vi "Execute_Row.vi"(3 "Simulate/Run":T2, 5 "Traverse line":T3 {"Carrier_2 Q (l/min)" format="%#.2f"; "Row Duration (mins)" format="%#.1f"; "Row No" min=0; "Trace Gas Concentration (%)" min=0.0 format="%#_4f"; "Carrier_1 Q (l/min)" format="%#.4f"; "Start X" format="%#.2f"; "Start Y" format="%#.2f"; "Start Z" format="%#.2f"; "End X" format="%#.2f"; "End Y" format="%#.2f"; "End Z" format="%#.2f"; "Tunnel Speed" format="%#.2f"; "Averaging time (mins)" min=0.0 format="%#.2f"}) -> (1 "Status":T1, 2 "Traverse line out":T3 {"Carrier_2 Q (l/min)" format="%#.2f"; "Row Duration (mins)" format="%#.1f"; "Row No" min=0; "Trace Gas Concentration (%)" min=0.0 format="%#_4f"; "Carrier_1 Q (l/min)" format="%#.4f"; "Start X" format="%#.2f"; "Start Y" format="%#.2f"; "Start Z" format="%#.2f"; "End X" format="%#.2f"; "End Y" format="%#.2f"; "End Z" format="%#.2f"; "Tunnel Speed" format="%#.2f"; "Averaging time (mins)" min=0.0 format="%#.2f"})   [LabVIEW 2021]
uses:
  Traverse_cluster.ctl
  Spacing.ctl
  Controls/Multi_run_mode.ctl
  Controls/User_Specific_mode.ctl
  Multi_Run_Status.ctl
  Controls/Setup.ctl
  Controls/Save_Data.ctl
  Camera Server/Camera enum/Camera resolution.ctl
  ADAM Client/Sub VIs/ADAM Controls/Quick_local_ADAM_Table.ctl
  Globals/Constants_global.vi
  Globals/Extra_Commands_Global.vi
  Globals/Trav_pos_global.vi
panel:
  # "X           Y          Z"
  # "Start"
  # "End"
  # "X           Y          Z"
  # "Start"
  # "End"
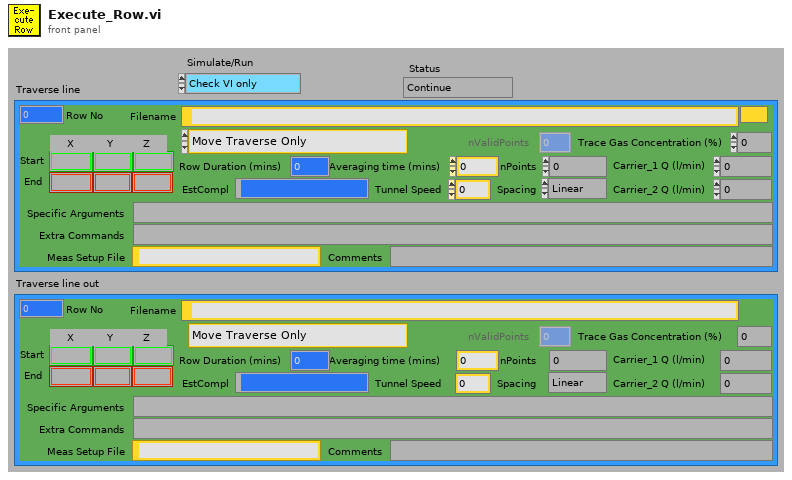
[diagram p1: front panel]
types:
  T1 = typedef "Multi_Run_Status.ctl" = enum16{"Continue", "Continue with Error", "Jump to Next Point", "Jump to Next Row", "Jump To Fall Back", "Terminate Run"}
  T2 = typedef "User_Specific_mode.ctl" = enum16{"Check VI only", "Run VI"}
  T3 = typedef "Traverse_cluster.ctl" = cluster{"Start X":sgl, "Start Y":sgl, "Start Z":sgl, "End X":sgl, "End Y":sgl, "End Z":sgl, "nPoints":i32, "Spacing":T4, "Filename":path, "Tunnel Speed":dbl, "Averaging time (mins)":dbl, "Extra Commands":string, "Carrier_1 Q (l/min)":dbl, "Carrier_2 Q (l/min)":dbl, "Trace Gas Concentration (%)":dbl, "Specific Arguments":string, "Comments":string, "Row No":i32, "Row Type Selector":T5, "EstCompl":string, "Row Duration (mins)":dbl, "nValidPoints":i32, "Meas Setup File":string}
  T4 = typedef "Spacing.ctl" = enum16{"Linear", "Log", "Gauss", "Specified", "N/A"}
  T5 = typedef "Multi_run_mode.ctl" = enum16{"Move Traverse Only", "Set Tunnel Speed Only", "Set Source Only", "Set Measurement Conditions", "Single Measurement", "Vertical Profile", "Lateral Profile", "Longitudinal Profile", "Multi-Axis Profile", "Explore Volume", "Auto Calibrate", "Meas Fast FID Bkgnd", "Check Beam Power", "Scanning Valve Measurement", "Run VI Named:", "Set ADAM Ch", "Wait (minutes)", "Send Message", "Synchronize With:", "Fall Back to this Row", "Turn Off Row Repeating", "Traverse 3D Volume", "Blank Row", "Jump to Fall Back Row"}
  T6 = typedef "Save_Data.ctl" = enum16{"Save No Data", "Save Data"}
  T7 = typedef "Setup.ctl" = enum16{"Run Program", "Show Setup", "Save Current Setup", "Setup Front Panel"}
  T8 = typedef "Quick_local_ADAM_Table.ctl" = enum16{"Read Global", "Load Global From ADAM Table", "Write Global"}
  T9 = typedef "Camera resolution.ctl" = u8
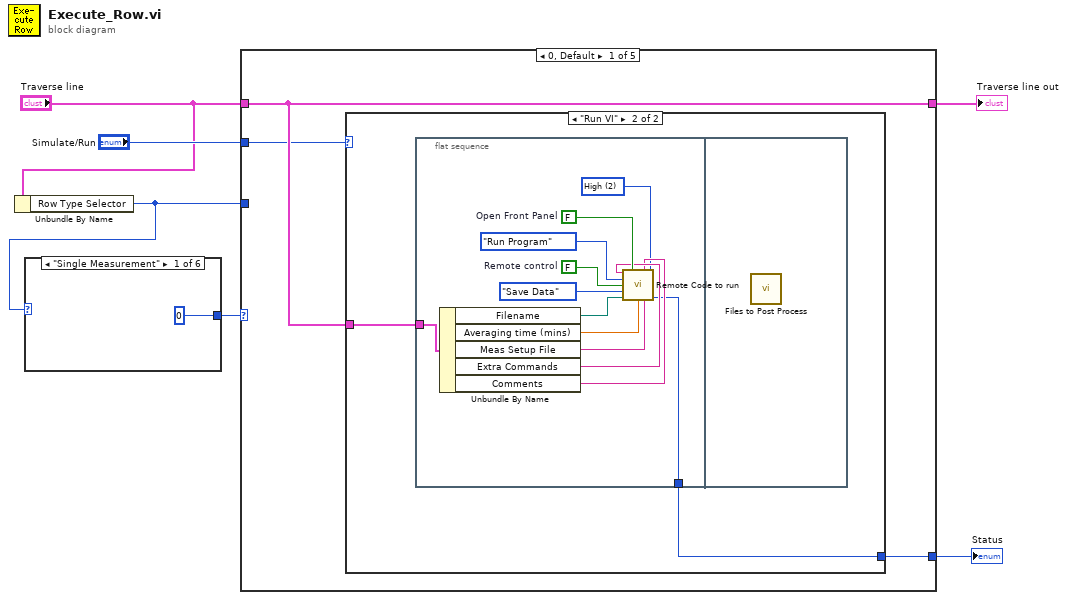
[diagram p0: block diagram]
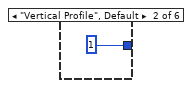
[diagram p2: hidden frame]
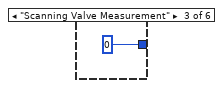
[diagram p3: hidden frame]
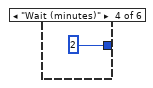
[diagram p4: hidden frame]
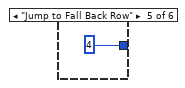
[diagram p5: hidden frame]
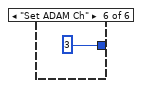
[diagram p6: hidden frame]
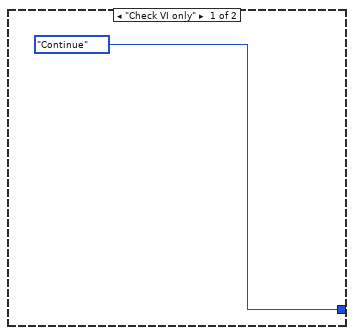
[diagram p7: hidden frame]
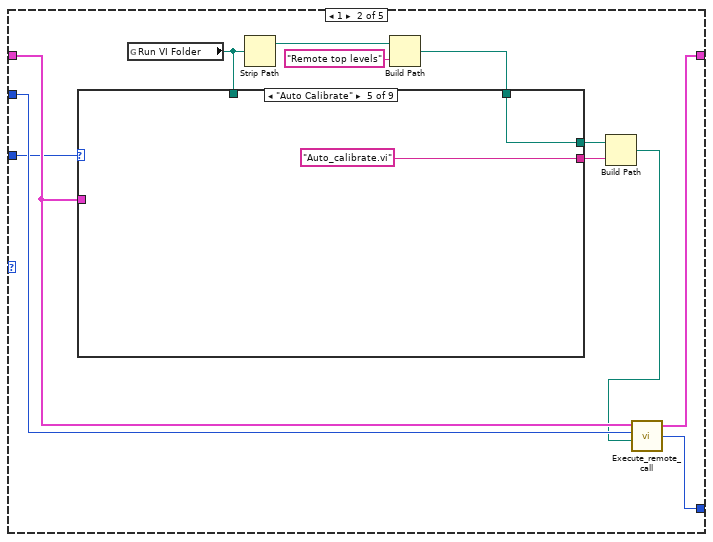
[diagram p8: hidden frame]
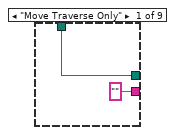
[diagram p9: hidden frame]
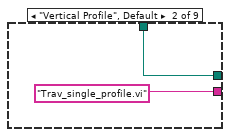
[diagram p10: hidden frame]
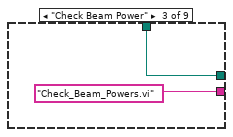
[diagram p11: hidden frame]
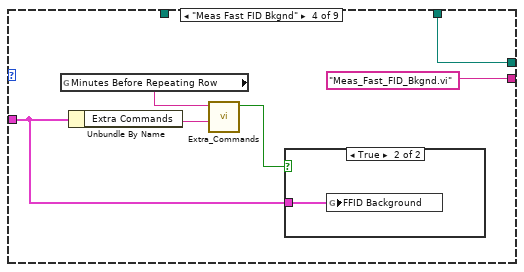
[diagram p12: hidden frame]
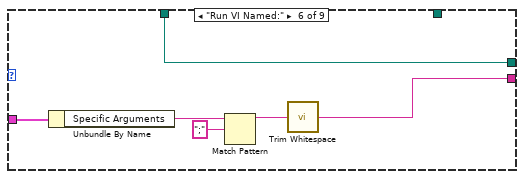
[diagram p14: hidden frame]
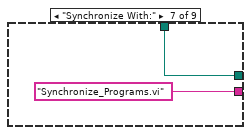
[diagram p15: hidden frame]
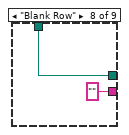
[diagram p16: hidden frame]
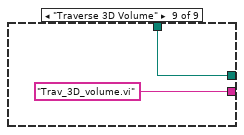
[diagram p17: hidden frame]
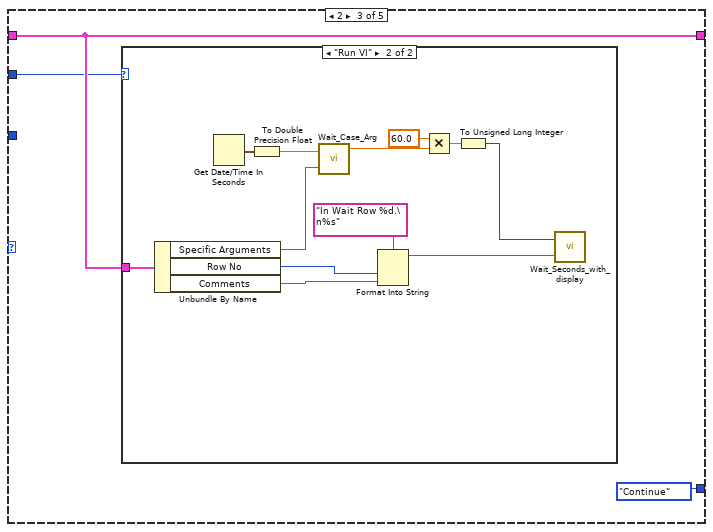
[diagram p18: hidden frame]
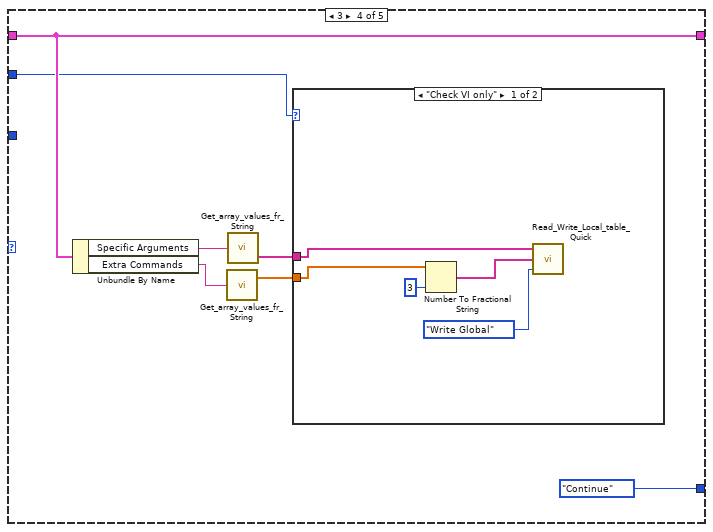
[diagram p20: hidden frame]
diagram:
  n1 = Unbundle By Name("Traverse line") -> ("Row Type Selector"=w2:T5)
  n2 = case shown="\"Single Measurement\"" w2 {
    tunnel: [0 1 0 2 4 3] -> w3
    frame "Single Measurement" {
    }
    frame "Vertical Profile", Default {
    }
    frame "Scanning Valve Measurement" {
    }
    frame "Wait (minutes)" {
    }
    frame "Jump to Fall Back Row" {
    }
    frame "Set ADAM Ch" {
    }
  }
  n3 = case shown="0, Default" w3 {
    tunnel: [w15 w38 Multi_Run_Status."Continue" ("Status") Multi_Run_Status."Continue" ("Status") w102] -> w1
    tunnel: "Traverse line" -> [w14 w40 w72 w90 w101]
    tunnel: [w14 w42 w72 w90 w101] -> w6
    tunnel: "Simulate/Run" -> [w13 w41 w70 w85 w100]
    tunnel: w2 -> [_ w39 _ _ _]
    frame 0, Default {
      n4 = case shown="\"Run VI\"" w13 {
        tunnel: [Multi_Run_Status."Continue" ("Status") w17] -> w15
        tunnel: w14 -> [_ w18]
        frame "Check VI only" {
        }
        frame "Run VI" {
          n5 = flat-sequence {
            tunnel: w18 -> [w30]
            tunnel: [w19] -> w17
            frame #0 {
              w20 = T9 2 items=["Low", "Med.", "High", "Max."] ("Camera Resolution")
              w26 = FALSE  # Open Front Panel
              w28 = FALSE  # Remote control
              n6 = Unbundle By Name(w30) -> ("Filename"=w29:path, "Averaging time (mins)"=w27:dbl, "Meas Setup File"=w23:string, "Extra Commands"=w22:string, "Comments"=w21:string)
              n7 = call "Remote Code to run.vi"("Extra command String"=w22, "Open Front Panel"=w26, "Current Row Comments"=w21, "Camera Resolution"=w20, "setup"=Setup."Run Program", "Remote control"=w28, "File"=Save_Data."Save Data", "Results Filename"=w29, "Averaging time (min)"=w27, "Setup filename"=w23) -> ("Status"=w19:T1)  [unwired: 5 in]
            }
            frame #1 {
              n8 = call "Files to Post Process.vi"() -> ()  [unwired: 12 in]
            }
          }
        }
      }
    }
    frame 1 {
      n9 = global read "Constants_global.vi" "Run VI Folder"() -> (w31:path)
      n10 = Strip Path(path=w31) -> (stripped path=w32:path)  [unwired: 1 out]
      n11 = Build Path(base path=w32, name or relative path="Remote top levels") -> (appended path=w36:path)
      n12 = case shown="\"Auto Calibrate\"" w39 {
        tunnel: w36 -> [w44 w46 w48 w54 w57 _ w65 w67 w69]
        tunnel: w40 -> [_ _ _ w49 _ w63 _ _ _]
        tunnel: [w44 w46 w48 w54 w57 w62 w65 w67 w69] -> w35
        tunnel: ["" ("name") "Trav_single_profile.vi" "Check_Beam_Powers.vi" "Meas_Fast_FID_Bkgnd.vi" "Auto_calibrate.vi" w58 "Synchronize_Programs.vi" "" ("name") "Trav_3D_volume.vi" ("name")] -> w34
        tunnel: w31 -> [_ _ _ _ _ w62 _ _ _]
        frame "Move Traverse Only" {
        }
        frame "Vertical Profile", Default {
        }
        frame "Check Beam Power" {
        }
        frame "Meas Fast FID Bkgnd" {
          n13 = global read "Extra_Commands_Global.vi" "Minutes Before Repeating Row"() -> (w52:string)
          n14 = Unbundle By Name(w49) -> ("Extra Commands"=w51:string)
          n15 = call "Extra_Commands.vi"("String to Search"=w51, "Command"=w52) -> ("Command Found"=w50:bool)  [unwired: 1 in, 4 out]
          n16 = case shown="True" w50 {
            tunnel: w49 -> [_ w55]
            frame False {
            }
            frame True {
              n17 = global write "Trav_pos_global.vi" "FFID Background"(w55) -> ()
            }
          }
        }
        frame "Auto Calibrate" {
        }
        frame "Run VI Named:" {
          n18 = Unbundle By Name(w63) -> ("Specific Arguments"=w60:string)
          n19 = Match Pattern(string=w60, regular expression=";") -> (before substring=w59:string)  [unwired: 4 out]
          n20 = call <vilib>:"Trim Whitespace.vi"("string"=w59) -> ("trimmed string"=w58:string)  [unwired: 1 in]
        }
        frame "Synchronize With:" {
        }
        frame "Blank Row" {
        }
        frame "Traverse 3D Volume" {
        }
      }
      n21 = Build Path(base path=w35, name or relative path=w34) -> (appended path=w33:path)
      n22 = call "Execute_remote_call.vi"("Traverse line"=w40, "Simulate/Run"=w41, "VI to run"=w33) -> ("Traverse Out"=w42:T3, "Status"=w38:T1)  [unwired: 1 in, 3 out]
    }
    frame 2 {
      n23 = case shown="\"Run VI\"" w70 {
        tunnel: w72 -> [_ w78]
        frame "Check VI only", Default {
        }
        frame "Run VI" {
          n24 = Unbundle By Name(w78) -> ("Specific Arguments"=w79:string, "Row No"=w74:i32, "Comments"=w73:string)
          n25 = Get Date/Time In Seconds() -> (seconds since 1Jan1904=w77:timestamp)
          n26 = To Double Precision Float(number=w77) -> (double precision float=w80:dbl)
          n27 = call "Wait_Case_Arg.vi"("Specific Argument"=w79, "seconds since 1Jan1904"=w80) -> ("Minutes To Wait"=w81:dbl)  [unwired: 4 out]
          n28 = Format Into String(format string="In Wait Row %d.\n%s", w74, w73) -> (resulting string=w76:string)  [unwired: 2 in, 1 out]
          n29 = Multiply(x=60.0, y=w81) -> (x*y=w82:dbl)
          n30 = To Unsigned Long Integer(number=w82) -> (unsigned 32bit integer=w83:u32)
          n31 = call "Wait_Seconds_with_display.vi"("Message"=w76, "Seconds to wait"=w83) -> ()  [unwired: 2 out]
        }
      }
    }
    frame 3 {
      n32 = Unbundle By Name(w90) -> ("Specific Arguments"=w89:string, "Extra Commands"=w87:string)
      n33 = call "Get_array_values_fr_String.vi"("String Value"=w87) -> ("Numeric Array"=w86:dbl[])  [unwired: 1 out]
      n34 = call "Get_array_values_fr_String.vi"("String Value"=w89) -> ("String array"=w88:string[])  [unwired: 1 out]
      n35 = case shown="\"Check VI only\"" w85 {
        tunnel: w88 -> [w92 w98]
        tunnel: w86 -> [w94 w97]
        frame "Check VI only" {
          n36 = Number To Fractional String(number=w94, precision (6)=i16 3) -> (F-format string=w93:string[])  [unwired: 2 in]
          n37 = call "Read_Write_Local_table_Quick.vi"("Mode"=Quick_local_ADAM_Table."Write Global", "String Values In"=w93, "Ch names In"=w92) -> ()  [unwired: 3 out]
        }
        frame "Run VI" {
          w99 = TRUE  # Check Value is in the scan table?
          n38 = call "ASYNC_Adam_client.vi"("Values"=w97, "Check Value is in the scan table?"=w99, "Channel Names"=w98) -> ()  [unwired: 2 out]
        }
      }
    }
    frame 4 {
      n39 = case shown="\"Run VI\"" w100 {
        tunnel: [Multi_Run_Status."Continue" ("Status") Multi_Run_Status."Jump To Fall Back" ("Status")] -> w102
        frame "Check VI only" {
        }
        frame "Run VI" {
        }
      }
    }
  }
  "Traverse line out" <- w6
  "Status" <- w1
